vi "GOOPUtil_GarbageCollector.vi"(1 "Class Names":string[](array[string]), 5 "error in (no error)":errorcluster) -> (15 "Nr Of Killed Objects":i32, 19 "error out":errorcluster)   [LabVIEW 2020, in "GOOPUtility.lvlib"]
doc: "When executed, all GOOP objects of the specified classes will be delete by running the Destroy (the destructor) method. If class name array is empty, all GOOP objects remaining in memory will be deleted.\n\nTypically this VI is executed as the last step of the main application.\n\nThis is a collection of generic GOOP utility VIs. Please notice that it is important that the frontpanel of the Create, Destroy and GetObjectStatus is not removed when building an application."
uses:
  GOOPUtility.lvlib
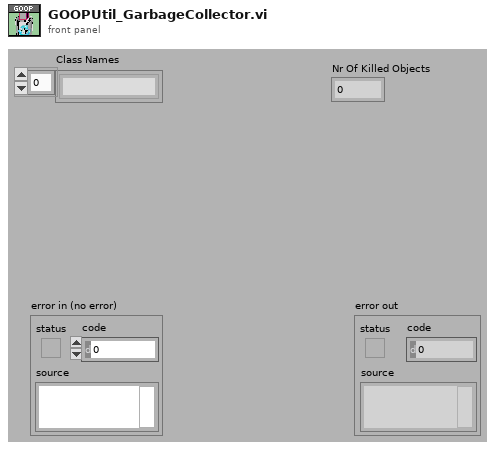
[diagram p1: front panel]
types:
  T1 = typedef "VIMemory VI info.ctl" = cluster{"Project":string, "ComputingNode":string, "VI Name":string, "App Refnum":refnum<vi>}
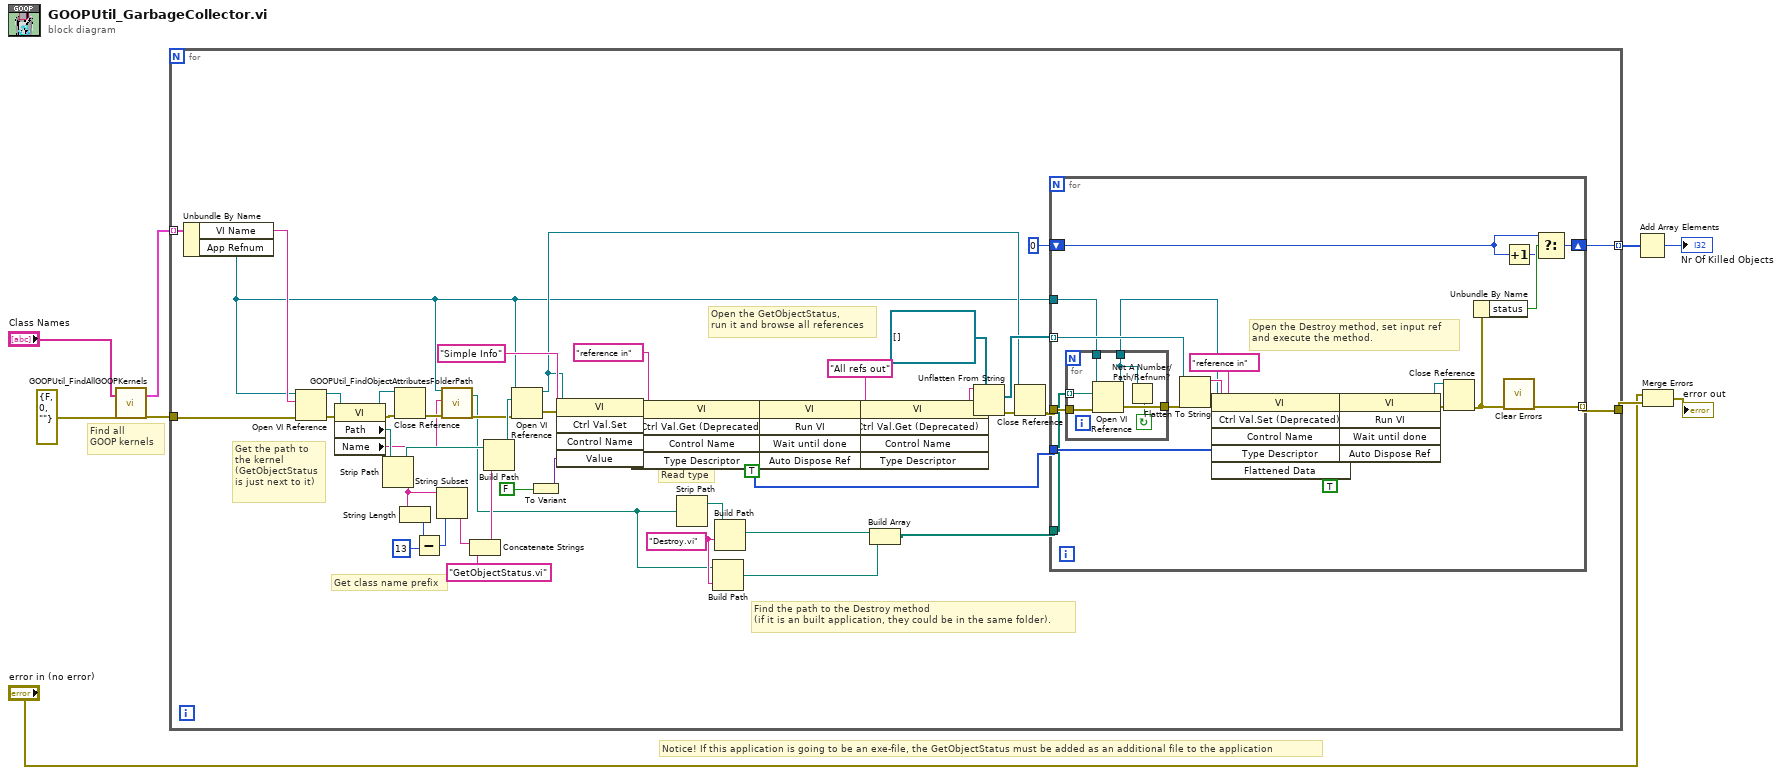
[diagram p0: block diagram]
diagram:
  # "Notice! If this application is going to be an exe-file, the GetObjectStatus must be added as an additional file to the application"
  # "Find all\nGOOP kernels"
  n1 = call "GOOPUtil_FindAllGOOPKernels.vi"("ClassNames"="Class Names", "error in (no error)"=errorcluster {"status"=FALSE, "code"=0, "source"=""}) -> ("GOOPKernels"=w8:T1[], "error out"=w9:errorcluster)  [unwired: 16 in]
  n2 = for {
    tunnel: w9 -> [w59]
    tunnel: w8 -> [w60] mode=indexing
    tunnel: [w42] -> w6
    tunnel: [w36] -> w4 mode=indexing
    w29 = "Destroy.vi"
    # "Get the path to\nthe kernel\n(GetObjectStatus\nis just next to it)"
    # "Find the path to the Destroy method\n(if it is an built application, they could be in the same folder)."
    # "Read type"
    # "Open the GetObjectStatus,\nrun it and browse all references"
    # "Get class name prefix"
    n3 = Unbundle By Name(w60) -> ("VI Name"=w58:string, "App Refnum"=w12:refnum<vi>)
    n4 = Open VI Reference(application reference (local)=w12, vi path=w58, error in (no error)=w59) -> (vi reference=w56:refnum<vi>, error out=w57:errorcluster)  [unwired: 3 in]
    n5 = property class="VI"(reference=w56, error in=w57) -> (reference out=w54:refnum<vi>, error out=w55:errorcluster, "Path"=w53:path, "Name"=w13:string)
    n6 = Strip Path(path=w53) -> (stripped path=w30:path, name=w49:string)
    n7 = Close Reference(reference=w54, error in (no error)=w55) -> (error out=w14:errorcluster)
    n8 = String Length(string=w49) -> (length=w52:i32)
    n9 = Subtract(x=w52, y=13) -> (x-y=w50:i32)
    n10 = String Subset(string=w49, length (rest)=w50) -> (substring=w44:string)  [unwired: 1 in]
    n11 = call "GOOPUtil_FindObjectAttributesFolderPath.vi"("application reference (local)"=w12, "GOOPKernelName"=w13, "error in (no error)"=w14) -> ("Folder"=w10:path, "error out"=w11:errorcluster)  [unwired: 15 in]
    n12 = Concatenate Strings(w44, "GetObjectStatus.vi") -> (w47:string)
    n13 = Build Path(base path=w30, name or relative path=w47) -> (appended path=w46:path)
    n14 = Open VI Reference(application reference (local)=w12, vi path=w46, error in (no error)=w11) -> (vi reference=w20:refnum<vi>, error out=w19:errorcluster)  [unwired: 3 in]
    n15 = To Variant(anything=FALSE ("Wait Until Done")) -> (Variant=w24:variant)
    n16 = invoke class="VI" method="Ctrl Val.Set"(reference=w20, error in=w19, "Control Name"="Simple Info", "Value"=w24) -> (reference out=w21:refnum<vi>, error out=w22:errorcluster)  [unwired: 1 in, 3 out]
    n17 = invoke class="VI" method="Ctrl Val.Get (Deprecated)"(reference=w21, error in=w22, "Control Name"="reference in") -> (reference out=w17:refnum<vi>, error out=w18:errorcluster, "Type Descriptor"=w38:i16[])  [unwired: 2 in, 2 out]
    n18 = Strip Path(path=w10) -> (stripped path=w41:path)  [unwired: 1 out]
    n19 = Build Path(base path=w10, name or relative path=w29) -> (appended path=w27:path)
    n20 = Build Path(base path=w41, name or relative path=w29) -> (appended path=w28:path)
    n21 = invoke class="VI" method="Run VI"(reference=w17, error in=w18, "Wait until done"=TRUE ("Wait Until Done")) -> (reference out=w16:refnum<vi>, error out=w15:errorcluster)  [unwired: 2 in, 3 out]
    n22 = invoke class="VI" method="Ctrl Val.Get (Deprecated)"(reference=w16, error in=w15, "Control Name"="All refs out") -> (error out=w35:errorcluster, "Get Control Value"=w33:string)  [unwired: 2 in, 3 out]
    n23 = Build Array(w28, w27) -> (w26:path[])
    n24 = Unflatten From String(type=refnum<class>[] [], binary string=w33, error in (no error)=w35) -> (value=w31:refnum<class>[], error out=w34:errorcluster)  [unwired: 2 in, 1 out]
    n25 = Close Reference(reference=w20, error in (no error)=w34) -> (error out=w43:errorcluster)
    n26 = for {
      tunnel: w26 -> [w62]
      tunnel: w43 -> [w76]
      tunnel: [w75] -> w42 mode=indexing
      tunnel: w38 -> [w73]
      shift-right: [w69] -> w36
      shift-left: 0 -> [w70]
      tunnel: w31 -> [w65] mode=indexing
      tunnel: w12 -> [w63]
      # "Open the Destroy method, set input ref\nand execute the method."
      n27 = for {
        tunnel: w76 -> [w87]
        tunnel: [w83] -> w61
        tunnel: [w86] -> w67
        tunnel: w63 -> [w85]
        tunnel: w62 -> [w84] mode=indexing
        stop <- w82 continue-if-true
        n28 = Open VI Reference(application reference (local)=w85, vi path=w84, error in (no error)=w87) -> (vi reference=w83:refnum<vi>, error out=w86:errorcluster)  [unwired: 3 in]
        n29 = Not A Number/Path/Refnum?(number/path/refnum=w83) -> (NaN/Path/Refnum?=w82:bool)
      }
      n30 = Flatten To String(anything=w65, error in (no error)=w67) -> (data string=w64:string, error out=w66:errorcluster)  [unwired: 2 in, 1 out]
      n31 = invoke class="VI" method="Ctrl Val.Set (Deprecated)"(reference=w61, error in=w66, "Control Name"="reference in", "Type Descriptor"=w73, "Flattened Data"=w64) -> (reference out=w79:refnum<vi>, error out=w80:errorcluster)  [unwired: 1 in, 4 out]
      n32 = invoke class="VI" method="Run VI"(reference=w79, error in=w80, "Wait until done"=TRUE ("Wait Until Done")) -> (reference out=w77:refnum<vi>, error out=w78:errorcluster)  [unwired: 2 in, 3 out]
      n33 = Close Reference(reference=w77, error in (no error)=w78) -> (error out=w68:errorcluster)
      n34 = Unbundle By Name(w68) -> ("status"=w72:bool)
      n35 = Increment(x=w70) -> (x+1=w71:i32)
      n36 = call <vilib>:"Clear Errors.vi"("error in (no error)"=w68) -> ("error out"=w75:errorcluster)  [unwired: 5 in, 1 out]
      n37 = Select(t=w70, s=w72, f=w71) -> (s? t:f=w69:i32)
    }
  }
  n38 = Add Array Elements(numeric array=w4) -> (sum=→"Nr Of Killed Objects":i32)
  n39 = Merge Errors("error in (no error)", w6) -> (→"error out":errorcluster)
